vi "上传数据.vi"(9 "标定站地址":u32=1 format="%x", 10 "初始地址":u32=15360 format="%x", 11 "多列列表框":refnum<vi>) -> (2 "输出数组":T1(array[cluster]))   [LabVIEW 2016]
panel:
  out "x != 0?":bool
  out "值":i32
  out "数组":u8[](array[numeric])
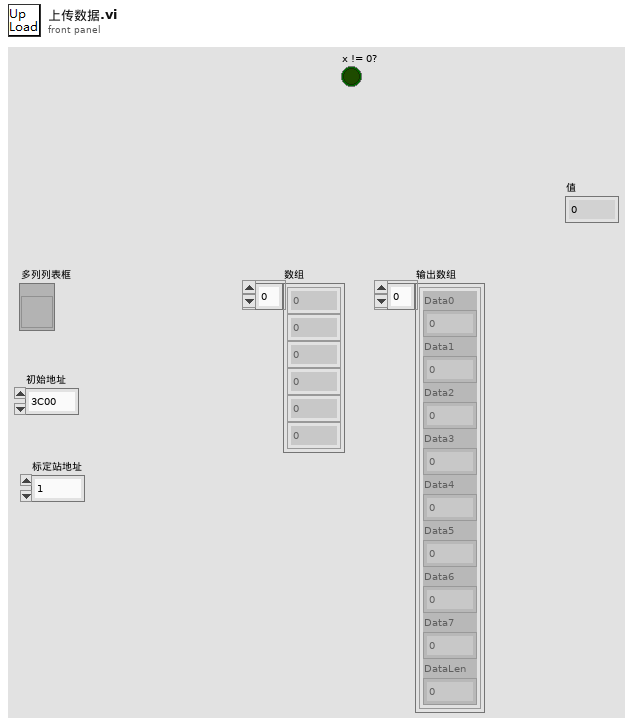
[diagram p1: front panel]
types:
  T1 = cluster{"Data0":u8, "Data1":u8, "Data2":u8, "Data3":u8, "Data4":u8, "Data5":u8, "Data6":u8, "Data7":u8, "DataLen":u8}[]
  T2 = cluster{"Data0":u8, "Data1":u8, "Data2":u8, "Data3":u8, "Data4":u8, "Data5":u8, "Data6":u8, "Data7":u8, "DataLen":u8}
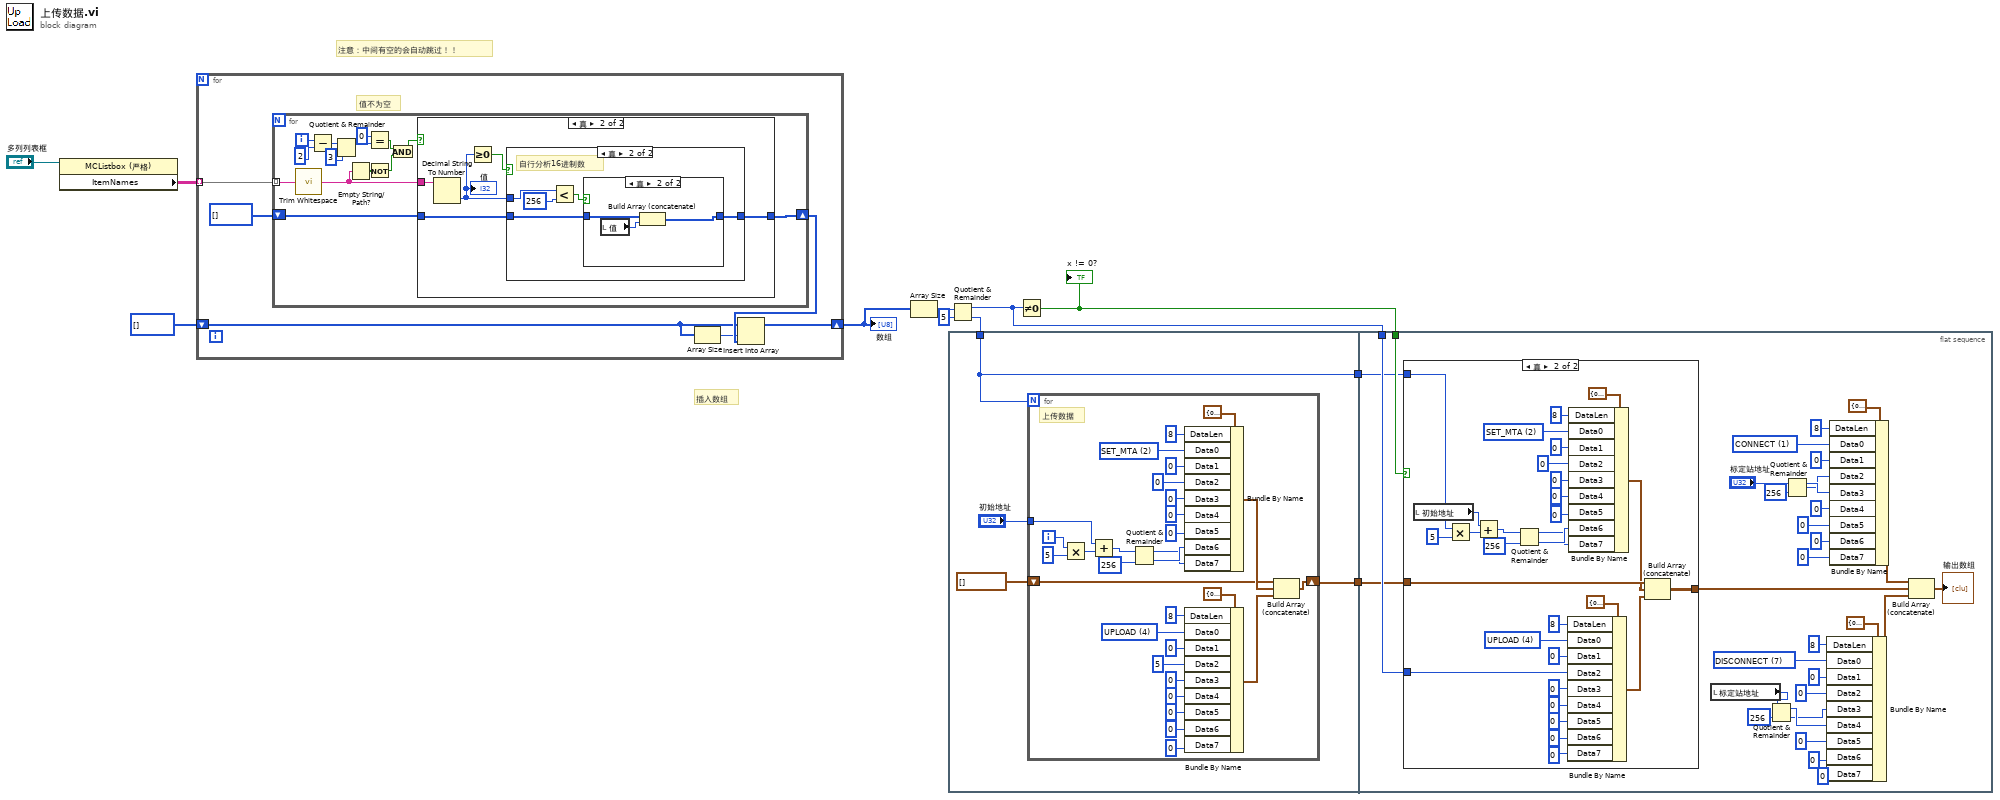
[diagram p0: block diagram]
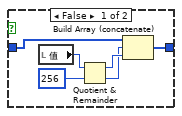
[diagram p5: hidden frame]
diagram:
  # "注意：中间有空的会自动跳过！！"
  # "插入数组"
  n1 = property class="MCListbox (严格)"(reference="多列列表框") -> ("ItemNames"=w9:string[][])  [unwired: 1 in, 2 out]
  n2 = for {
    tunnel: w9 -> [w17] mode=indexing
    shift-right: [w12] -> w8
    shift-left: i32[] [] -> [w14]
    # "值不为空"
    n3 = for {
      tunnel: w17 -> [w24] mode=indexing
      shift-right: [w23] -> w15
      shift-left: i32[] [] -> [w25]
      i -> [w31]
      n4 = call <vilib>:"Trim Whitespace.vi"("string"=w24) -> ("trimmed string"=w22:string)  [unwired: 1 in]
      n5 = Subtract(x=w31, y=2) -> (x-y=w29:i32)
      n6 = Quotient & Remainder(x=w29, y=3) -> (x-y*floor(x/y)=w27:i32)  [unwired: 1 out]
      n7 = Empty String/Path?(string/path=w22) -> (empty?=w21:bool)
      n8 = Equal?(x=0, y=w27) -> (x = y?=w19:bool)
      n9 = Not(x=w21) -> (.not. x?=w20:bool)
      n10 = And(x=w19, y=w20) -> (x .and. y?=w18:bool)
      n11 = case shown="真" w18 {
        tunnel: w22 -> [_ w37]
        tunnel: w25 -> [w32 w34]
        tunnel: [w32 w33] -> w23
        frame False {
        }
        frame True {
          n12 = Decimal String To Number(string=w37) -> (number=w35:i32)  [unwired: 2 in, 1 out]
          "值" <- w35
          n13 = Greater Or Equal To 0?(x=w35) -> (x >= 0?=w36:bool)
          n14 = case shown="真" w36 {
            tunnel: w35 -> [_ w43]
            tunnel: [w38 w40] -> w33
            tunnel: w34 -> [w38 w39]
            frame False {
            }
            frame True {
              # "自行分析16进制数"
              n15 = Less?(x=w43, y=256) -> (x < y?=w41:bool)
              n16 = case shown="真" w41 {
                tunnel: [w49 w50] -> w40
                tunnel: w39 -> [w48 w52]
                frame False {
                  n17 = local read "值"() -> (w47:i32)
                  n18 = Quotient & Remainder(x=w47, y=256) -> (x-y*floor(x/y)=w45:i32, floor(x/y)=w44:i32)
                  n19 = Build Array (concatenate)(w48, w44, w45) -> (w49:i32[])
                }
                frame True {
                  n20 = local read "值"() -> (w51:i32)
                  n21 = Build Array (concatenate)(w52, w51) -> (w50:i32[])
                }
              }
            }
          }
        }
      }
    }
    n22 = Array Size(array=w14) -> (size(s)=w13:i32)
    n23 = Insert Into Array(array=w14, index=w13, new element=w15) -> (w12:i32[])
  }
  "数组" <- w8
  n24 = Array Size(array=w8) -> (size(s)=w7:i32)
  n25 = flat-sequence {
    tunnel: w5 -> [w53]
    tunnel: [w54] -> w4
    tunnel: [w53] -> w1
    tunnel: w4 -> [w116]
    tunnel: w3 -> [w118]
    tunnel: w2 -> [w117]
    tunnel: w1 -> [w115]
    frame #0 {
      n26 = for {
        N: w53 -> [_]
        tunnel: "初始地址" -> [w59]
        shift-right: [w58] -> w54
        shift-left: T1 [] -> [w57]
        i -> [w60]
        w68 = u16 2 items=["CONNECT"=1, "SET_MTA"=2, "DNLOAD"=3, "UPLOAD"=4, "DISCONNECT"=7, "START_STOP_ALL"=8, "SHORT_UPLOAD"=15, "GET_DAQ_SIZE"=20, "SET_DAQ_PTR"=21, "WRITE_DAQ"=22, "EXCHANGE_ID"=23, "DNLOAD6"=35, "UNLOACK"=19, "SET_S_STATUS"=12, "GET_S_STATUS"=13, "SET_CAL_PAGE"=17, "GET_CAL_PAGE"=9, "GET_SEED"=18] ("下拉列表")
        w67 = u16 4 items=["CONNECT"=1, "SET_MTA"=2, "DNLOAD"=3, "UPLOAD"=4, "DISCONNECT"=7, "START_STOP_ALL"=8, "SHORT_UPLOAD"=15, "GET_DAQ_SIZE"=20, "SET_DAQ_PTR"=21, "WRITE_DAQ"=22, "EXCHANGE_ID"=23, "DNLOAD6"=35, "UNLOACK"=19, "SET_S_STATUS"=12, "GET_S_STATUS"=13, "SET_CAL_PAGE"=17, "GET_CAL_PAGE"=9, "GET_SEED"=18] ("下拉列表")
        # "上传数据"
        n27 = Multiply(x=w60, y=5) -> (x*y=w81:i32)
        n28 = Add(x=w59, y=w81) -> (x+y=w80:u32)
        n29 = Quotient & Remainder(x=w80, y=u32 256) -> (x-y*floor(x/y)=w72:u32, floor(x/y)=w73:u32)
        n30 = Bundle By Name(cluster=T2 {"Data0"=0, "Data1"=0, "Data2"=0, "Data3"=0, "Data4"=0, "Data5"=0, "Data6"=0, "Data7"=0, "DataLen"=8} ("簇 2"), "DataLen"=u8 8, "Data0"=w68, "Data1"=u8 0, "Data2"=u8 0, "Data3"=u8 0, "Data4"=u8 0, "Data5"=u8 0, "Data6"=w73, "Data7"=w72) -> (w69:T2)
        n31 = Bundle By Name(cluster=T2 {"Data0"=0, "Data1"=0, "Data2"=0, "Data3"=0, "Data4"=0, "Data5"=0, "Data6"=0, "Data7"=0, "DataLen"=8} ("簇 2"), "DataLen"=u8 8, "Data0"=w67, "Data1"=u8 0, "Data2"=u8 5, "Data3"=u8 0, "Data4"=u8 0, "Data5"=u8 0, "Data6"=u8 0, "Data7"=u8 0) -> (w83:T2)
        n32 = Build Array (concatenate)(w57, w69, w83) -> (w58:T1)
      }
    }
    frame #1 {
      w100 = u8 7 items=["CONNECT"=1, "SET_MTA"=2, "DNLOAD"=3, "UPLOAD"=4, "DISCONNECT"=7, "START_STOP_ALL"=8, "SHORT_UPLOAD"=15, "GET_DAQ_SIZE"=20, "SET_DAQ_PTR"=21, "WRITE_DAQ"=22, "EXCHANGE_ID"=23, "DNLOAD6"=35, "UNLOACK"=19, "SET_S_STATUS"=12, "GET_S_STATUS"=13, "SET_CAL_PAGE"=17, "GET_CAL_PAGE"=9, "GET_SEED"=18] ("下拉列表")
      w112 = u8 1 items=["CONNECT"=1, "SET_MTA"=2, "DNLOAD"=3, "UPLOAD"=4, "DISCONNECT"=7, "START_STOP_ALL"=8, "SHORT_UPLOAD"=15, "GET_DAQ_SIZE"=20, "SET_DAQ_PTR"=21, "WRITE_DAQ"=22, "EXCHANGE_ID"=23, "DNLOAD6"=35, "UNLOACK"=19, "SET_S_STATUS"=12, "GET_S_STATUS"=13, "SET_CAL_PAGE"=17, "GET_CAL_PAGE"=9, "GET_SEED"=18] ("下拉列表")
      n33 = case shown="真" w118 {
        tunnel: w117 -> [_ w140]
        tunnel: w116 -> [w119 w139]
        tunnel: [w119 w138] -> w88
        tunnel: w115 -> [_ w121]
        frame False {
        }
        frame True {
          w124 = u16 2 items=["CONNECT"=1, "SET_MTA"=2, "DNLOAD"=3, "UPLOAD"=4, "DISCONNECT"=7, "START_STOP_ALL"=8, "SHORT_UPLOAD"=15, "GET_DAQ_SIZE"=20, "SET_DAQ_PTR"=21, "WRITE_DAQ"=22, "EXCHANGE_ID"=23, "DNLOAD6"=35, "UNLOACK"=19, "SET_S_STATUS"=12, "GET_S_STATUS"=13, "SET_CAL_PAGE"=17, "GET_CAL_PAGE"=9, "GET_SEED"=18] ("下拉列表")
          w146 = u16 4 items=["CONNECT"=1, "SET_MTA"=2, "DNLOAD"=3, "UPLOAD"=4, "DISCONNECT"=7, "START_STOP_ALL"=8, "SHORT_UPLOAD"=15, "GET_DAQ_SIZE"=20, "SET_DAQ_PTR"=21, "WRITE_DAQ"=22, "EXCHANGE_ID"=23, "DNLOAD6"=35, "UNLOACK"=19, "SET_S_STATUS"=12, "GET_S_STATUS"=13, "SET_CAL_PAGE"=17, "GET_CAL_PAGE"=9, "GET_SEED"=18] ("下拉列表")
          n34 = local read "初始地址"() -> (w120:u32)
          n35 = Multiply(x=w121, y=5) -> (x*y=w136:i32)
          n36 = Add(x=w120, y=w136) -> (x+y=w135:u32)
          n37 = Quotient & Remainder(x=w135, y=u32 256) -> (x-y*floor(x/y)=w127:u32, floor(x/y)=w128:u32)
          n38 = Bundle By Name(cluster=T2 {"Data0"=0, "Data1"=0, "Data2"=0, "Data3"=0, "Data4"=0, "Data5"=0, "Data6"=0, "Data7"=0, "DataLen"=8} ("簇 2"), "DataLen"=u8 8, "Data0"=w146, "Data1"=u8 0, "Data2"=w140, "Data3"=u8 0, "Data4"=u8 0, "Data5"=u8 0, "Data6"=u8 0, "Data7"=u8 0) -> (w122:T2)
          n39 = Bundle By Name(cluster=T2 {"Data0"=0, "Data1"=0, "Data2"=0, "Data3"=0, "Data4"=0, "Data5"=0, "Data6"=0, "Data7"=0, "DataLen"=8} ("簇 2"), "DataLen"=u8 8, "Data0"=w124, "Data1"=u8 0, "Data2"=u8 0, "Data3"=u8 0, "Data4"=u8 0, "Data5"=u8 0, "Data6"=w128, "Data7"=w127) -> (w123:T2)
          n40 = Build Array (concatenate)(w139, w123, w122) -> (w138:T1)
        }
      }
      n41 = local read "标定站地址"() -> (w89:u32)
      n42 = Quotient & Remainder(x=w89, y=u32 256) -> (x-y*floor(x/y)=w91:u32, floor(x/y)=w90:u32)
      n43 = Quotient & Remainder(x="标定站地址", y=u32 256) -> (x-y*floor(x/y)=w104:u32, floor(x/y)=w103:u32)
      n44 = Bundle By Name(cluster=T2 {"Data0"=0, "Data1"=0, "Data2"=0, "Data3"=0, "Data4"=0, "Data5"=0, "Data6"=0, "Data7"=0, "DataLen"=8} ("簇 2"), "DataLen"=u8 8, "Data0"=w100, "Data1"=u8 0, "Data2"=u8 0, "Data3"=w90, "Data4"=w91, "Data5"=u8 0, "Data6"=u8 0, "Data7"=u8 0) -> (w93:T2)
      n45 = Bundle By Name(cluster=T2 {"Data0"=0, "Data1"=0, "Data2"=0, "Data3"=0, "Data4"=0, "Data5"=0, "Data6"=0, "Data7"=0, "DataLen"=8} ("簇 2"), "DataLen"=u8 8, "Data0"=w112, "Data1"=u8 0, "Data2"=w103, "Data3"=w104, "Data4"=u8 0, "Data5"=u8 0, "Data6"=u8 0, "Data7"=u8 0) -> (w94:T2)
      n46 = Build Array (concatenate)(w94, w88, w93) -> (→"输出数组":T1)
    }
  }
  n47 = Quotient & Remainder(x=w7, y=5) -> (x-y*floor(x/y)=w2:i32, floor(x/y)=w5:i32)
  n48 = Not Equal To 0?(x=w2) -> (x != 0?=w3:bool)
  "x != 0?" <- w3
